vi "DT_Triangle Manager_Resize.vi"(10 "# of triangles":i32, 11 "Triangles In":i32[][](array[numeric])) -> (3 "Triangles Out":i32[][](array[numeric]))   [LabVIEW 2020, in "NI_AAL_Geometry.lvlib"]
uses:
  <vilib>/Analysis/NI_AAL_Geometry.lvlib
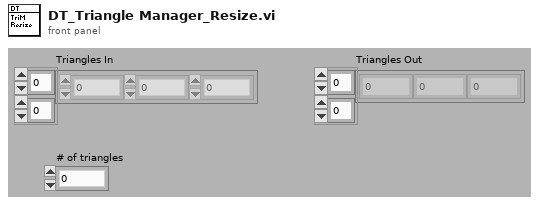
[diagram p1: front panel]
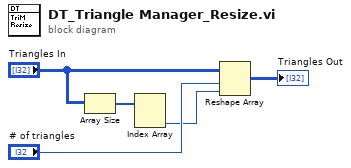
[diagram p0: block diagram]
diagram:
  n1 = Array Size(array="Triangles In") -> (size(s)=w2:i32[])
  n2 = Index Array(array=w2) -> (element #2=w1:i32)  [unwired: 2 in, 1 out]
  n3 = Reshape Array("Triangles In", "# of triangles", w1) -> (→"Triangles Out":i32[][])
